vi "Diplay_TestList.vi"(8 "error in (no error)":errorcluster, 9 "Descripbe":string="Start test", 11 "Limit input":string="CH116~1.2~1.6") -> (0 "error out":errorcluster={"status"=TRUE, "code"=-1073807343, "source"="Property Node (arg 1) in VISA Configure Serial Port (Instr).vi->ReadChanel.vi->CheckTestStart.vi"}, 1 "TestData":string="0.000000-----0.000000", 2 "TestResult":bool, 3 "Limit out":string="1.2------1.6", 4 "Descripbe output":string="Start test   (CH116)")   [LabVIEW 2013]
uses:
  <vilib>/Utility/error.llb/whitespace.ctl
  MainProgram/Control/Buffer.vi
panel:
  out "number":dbl
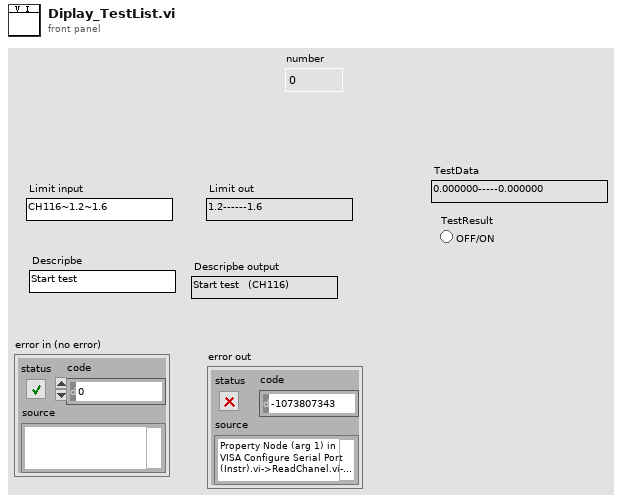
[diagram p1: front panel]
types:
  T1 = typedef "whitespace.ctl" = u16
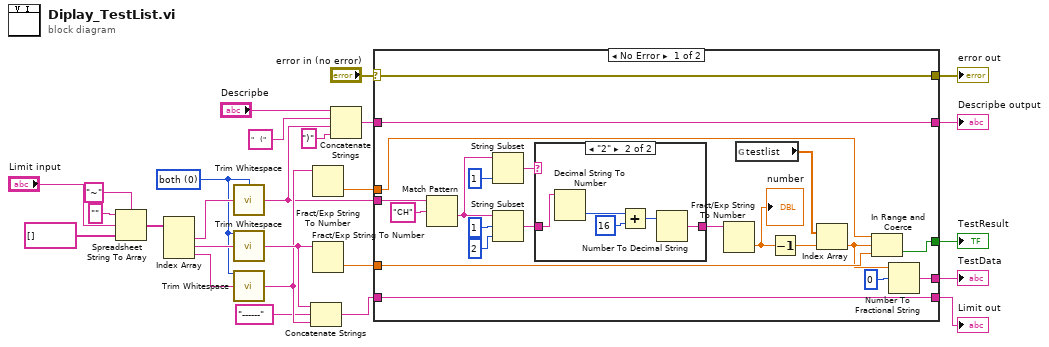
[diagram p0: block diagram]
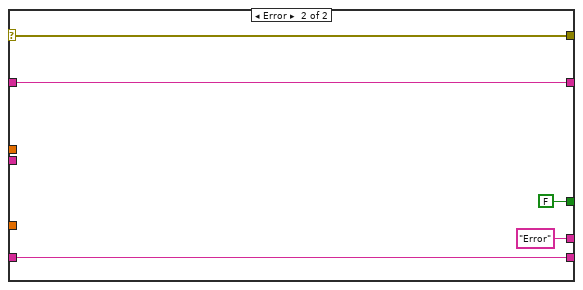
[diagram p3: hidden frame]
diagram:
  w18 = T1 0 items=["both", "start of string", "end of string"] ("location (both)")
  n1 = Spreadsheet String To Array(delimiter (Tab)="~", format string="", spreadsheet string="Limit input", array type (2D Dbl)=string[] []) -> (array=w22:string[])
  n2 = Index Array(array=w22) -> (element #1=w21:string, element #2=w20:string, element #3=w19:string)  [unwired: 3 in]
  n3 = call <vilib>:"Trim Whitespace.vi"("string"=w21, "location (both)"=w18) -> ("trimmed string"=w4:string)
  n4 = call <vilib>:"Trim Whitespace.vi"("string"=w20, "location (both)"=w18) -> ("trimmed string"=w13:string)
  n5 = call <vilib>:"Trim Whitespace.vi"("string"=w19, "location (both)"=w18) -> ("trimmed string"=w12:string)
  n6 = Concatenate Strings(w13, "------" ("string"), w12) -> (w9:string)
  n7 = Fract/Exp String To Number(string=w12) -> (number=w15:dbl)  [unwired: 3 in, 1 out]
  n8 = Fract/Exp String To Number(string=w13) -> (number=w17:dbl)  [unwired: 3 in, 1 out]
  n9 = Concatenate Strings("Descripbe", "   (" ("string"), w4, ")" ("string")) -> (w3:string)
  n10 = case shown="No Error" "error in (no error)" {
    selector: "error in (no error)" -> [w36 w58]
    tunnel: [w36 w58] -> w1
    tunnel: w4 -> [w45 _]
    tunnel: w17 -> [w42 _]
    tunnel: [w41 FALSE] -> w16
    tunnel: w15 -> [w43 _]
    tunnel: [w46 w56] -> w10
    tunnel: w9 -> [w46 w56]
    tunnel: [w44 w55] -> w8
    tunnel: w3 -> [w44 w55]
    tunnel: [w39 "Error" ("read buffer")] -> w2
    frame No Error {
      n11 = Match Pattern(string=w45, regular expression="CH") -> (after substring=w28:string)  [unwired: 1 in, 3 out]
      n12 = String Subset(string=w28, length (rest)=1 ("length (rest)")) -> (substring=w30:string)  [unwired: 1 in]
      n13 = String Subset(string=w28, offset (0)=1, length (rest)=2 ("length (rest)")) -> (substring=w29:string)
      n14 = case shown="\"2\"" w30 {
        tunnel: w29 -> [w48 w53]
        tunnel: [w48 w49] -> w27
        frame "1", Default {
        }
        frame "2" {
          n15 = Decimal String To Number(string=w53) -> (number=w52:i32)  [unwired: 2 in, 1 out]
          n16 = Add(x=w52, y=16) -> (x+y=w50:i32)
          n17 = Number To Decimal String(number=w50) -> (decimal integer string=w49:string)  [unwired: 1 in]
        }
      }
      n18 = Fract/Exp String To Number(string=w27) -> (number=w38:dbl)  [unwired: 3 in, 1 out]
      "number" <- w38
      n19 = global read "Buffer.vi" "testlist"() -> (w40:dbl[])
      n20 = Decrement(x=w38) -> (x-1=w34:dbl)
      n21 = Index Array(array=w40, index=w34) -> (element=w37:dbl)
      n22 = In Range and Coerce(upper limit=w43, x=w37, lower limit=w42) -> (In Range?=w41:bool)  [unwired: 1 out]
      n23 = Number To Fractional String(number=w37, width (-)=i16 0) -> (F-format string=w39:string)  [unwired: 2 in]
    }
    frame Error {
    }
  }
  "error out" <- w1
  "TestResult" <- w16
  "TestData" <- w2
  "Limit out" <- w10
  "Descripbe output" <- w8
